vi "start.vi"(10 "Parameters":T2, 11 "Cluster in":T1) -> (3 "Cluster out":T3)   [LabVIEW 2015]
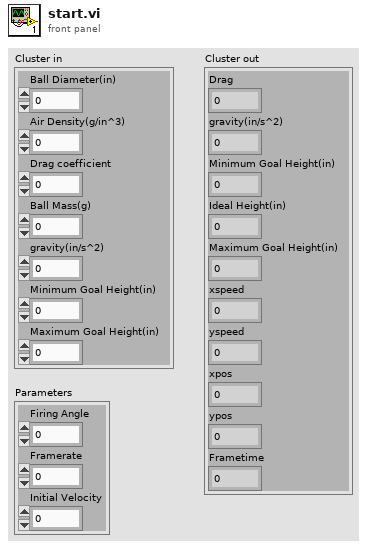
[diagram p1: front panel]
types:
  T1 = cluster{"Ball Diameter(in)":dbl, "Air Density(g/in^3)":dbl, "Drag coefficient":dbl, "Ball Mass(g)":dbl, "gravity(in/s^2)":dbl, "Minimum Goal Height(in)":dbl, "Maximum Goal Height(in)":dbl}
  T2 = cluster{"Firing Angle":dbl, "Framerate":dbl, "Initial Velocity":dbl}
  T3 = cluster{"Drag":dbl, "gravity(in/s^2)":dbl, "Minimum Goal Height(in)":dbl, "Ideal Height(in)":dbl, "Maximum Goal Height(in)":dbl, "xspeed":dbl, "yspeed":dbl, "xpos":dbl, "ypos":dbl, "Frametime":dbl}
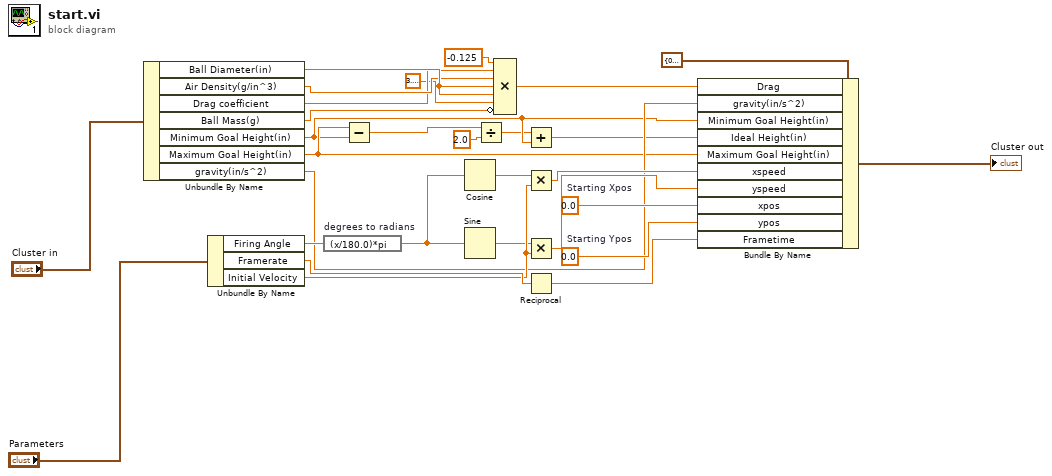
[diagram p0: block diagram]
diagram:
  w28 = 0.0  # Starting Xpos
  w29 = 0.0  # Starting Ypos
  n1 = Unbundle By Name("Cluster in") -> ("Ball Diameter(in)"=w11:dbl, "Air Density(g/in^3)"=w9:dbl, "Drag coefficient"=w8:dbl, "Ball Mass(g)"=w10:dbl, "Minimum Goal Height(in)"=w17:dbl, "Maximum Goal Height(in)"=w18:dbl, "gravity(in/s^2)"=w19:dbl)
  n2 = Unbundle By Name("Parameters") -> ("Firing Angle"=w23:dbl, "Framerate"=w22:dbl, "Initial Velocity"=w21:dbl)
  n3 = expression code="(x/180.0)*pi" "degrees to radians"(w23) -> (w13:dbl)
  n4 = Subtract(x=w18, y=w17) -> (x-y=w4:dbl)
  n5 = Cosine(x=w13) -> (cos(x)=w2:dbl)
  n6 = Sine(x=w13) -> (sin(x)=w1:dbl)
  n7 = Divide(x=w4, y=2.0) -> (x/y=w5:dbl)
  n8 = Compound Arithmetic op=MULTIPLY(-0.125 ("value"), w8, w9, w11, w11, 3.141592653589793, invert w10) -> (w20:dbl)
  n9 = Add(x=w5, y=w17) -> (x+y=w16:dbl)
  n10 = Multiply(x=w2, y=w21) -> (x*y=w26:dbl)
  n11 = Multiply(x=w1, y=w21) -> (x*y=w25:dbl)
  n12 = Reciprocal(x=w22) -> (1/x=w27:dbl)
  n13 = Bundle By Name(cluster=T3 {"Drag"=0.0, "gravity(in/s^2)"=-386.09, "Minimum Goal Height(in)"=85.0, "Ideal Height(in)"=0.0, "Maximum Goal Height(in)"=109.0, "xspeed"=0.0, "yspeed"=0.0, "xpos"=0.0, "ypos"=0.0, "Frametime"=0.0}, "Drag"=w20, "gravity(in/s^2)"=w19, "Minimum Goal Height(in)"=w17, "Ideal Height(in)"=w16, "Maximum Goal Height(in)"=w18, "xspeed"=w26, "yspeed"=w25, "xpos"=w28, "ypos"=w29, "Frametime"=w27) -> (→"Cluster out":T3)
